vi "setpoint(SubVI).vi"(0 "Filed 2":dbl=300.0, 1 "Field":dbl=300.0, 2 "类型":enum16{"temp", "field", "position"}(ring), 3 "Rate/speed":dbl=10.0, 4 "Mode":i32(ring) items=["Persistent", "Driven"], 5 "输出簇 2":T1={"initialize"="", "6221"={"6221 Resource"="GPIB0::24::INSTR", "Delta status"=FALSE}, "7001"={"Ch"=FALSE}, "SR830+6221"={"source"=0, "阻抗"=0.0, "量程入 4"=0, "量程入 3"=0, "量程入 2"=0, "量程入 1"=0, "电流"=0.0, "SR830 2"=FALSE, "SR830 3"=FALSE, "SR830 4"=FALSE, "SR830 1"=FALSE, "VISA 1"="", "VISA 2"="", "VISA 3"="", "VISA 4"="", "量程"=enum."量程每次测量会判定"}, "2400"={"2400"=FALSE, "VISA"=""}, "ch"={"ch"=[], "current"=[], "change?"=[]}, "log"={"log路径"=path "", "log interval"=0.0}, "Instrument"={"335 Resource"="GPIB0::24::INSTR", "Input (0:A)"=0, "Instrument Type"=3, "quantum design"=refnum, "Heater Output (1:1)"=1, "semaphore"=refnum, "TCP master instance"=refnum, "335 Status"=refnum, "M24C Resource"="GPIB0::24::INSTR", "4G supply"="GPIB0::24::INSTR", "Temp Status 24C"=refnum, "4g supply status"=refnum}, "Aborting"=refnum, "数据文件"=refnum} {"Instrument"."Input (0:A)" items=["A", "B"]; "Instrument"."Instrument Type" items=["PPMS", "VersaLab", "DynaCool", "SVSM", "Lakeshore335", "PPMS-Rotate"]; "Instrument"."Heater Output (1:1)" items=["1"=1, "2"=2]; "SR830+6221"."source" items=["SR830 1", "SR830 2", "SR830 3", "SR830 4"]}, 6 "data":refnum<queue>, 7 "Delay":dbl, 9 "steps number":i32, 11 "Approach":i32(ring) items=["FastSettle", "NoOvershoot"]) -> (8 "错误输出":errorcluster, 15 "输出簇":T1={"initialize"="", "6221"={"6221 Resource"="GPIB0::24::INSTR", "Delta status"=FALSE}, "7001"={"Ch"=FALSE}, "SR830+6221"={"source"=0, "阻抗"=0.0, "量程入 4"=0, "量程入 3"=0, "量程入 2"=0, "量程入 1"=0, "电流"=0.0, "SR830 2"=FALSE, "SR830 3"=FALSE, "SR830 4"=FALSE, "SR830 1"=FALSE, "VISA 1"="", "VISA 2"="", "VISA 3"="", "VISA 4"="", "量程"=enum."量程每次测量会判定"}, "2400"={"2400"=FALSE, "VISA"=""}, "ch"={"ch"=[], "current"=[], "change?"=[]}, "log"={"log路径"=path "", "log interval"=0.0}, "Instrument"={"335 Resource"="GPIB0::24::INSTR", "Input (0:A)"=0, "Instrument Type"=3, "quantum design"=refnum, "Heater Output (1:1)"=1, "semaphore"=refnum, "TCP master instance"=refnum, "335 Status"=refnum, "M24C Resource"="GPIB0::24::INSTR", "4G supply"="GPIB0::24::INSTR", "Temp Status 24C"=refnum, "4g supply status"=refnum}, "Aborting"=refnum, "数据文件"=refnum} {"Instrument"."Input (0:A)" items=["A", "B"]; "Instrument"."Instrument Type" items=["PPMS", "VersaLab", "DynaCool", "SVSM", "Lakeshore335", "PPMS-Rotate"]; "Instrument"."Heater Output (1:1)" items=["1"=1, "2"=2]; "SR830+6221"."source" items=["SR830 1", "SR830 2", "SR830 3", "SR830 4"]})   [LabVIEW 2019, in "SubVI.lvlib"]
uses:
  SubVI.lvlib
  config.ctl
  <vilib>/NI/Modbus Library/API/Master/Modbus Master.lvclass
  Instrument.ctl
  lib/QDInstrument.dll
  335 state.ctl
  9T cmag.lvlib
panel:
  # "(真是通道1，假是通道2)"
  # "(真是通道1，假是通道2)"
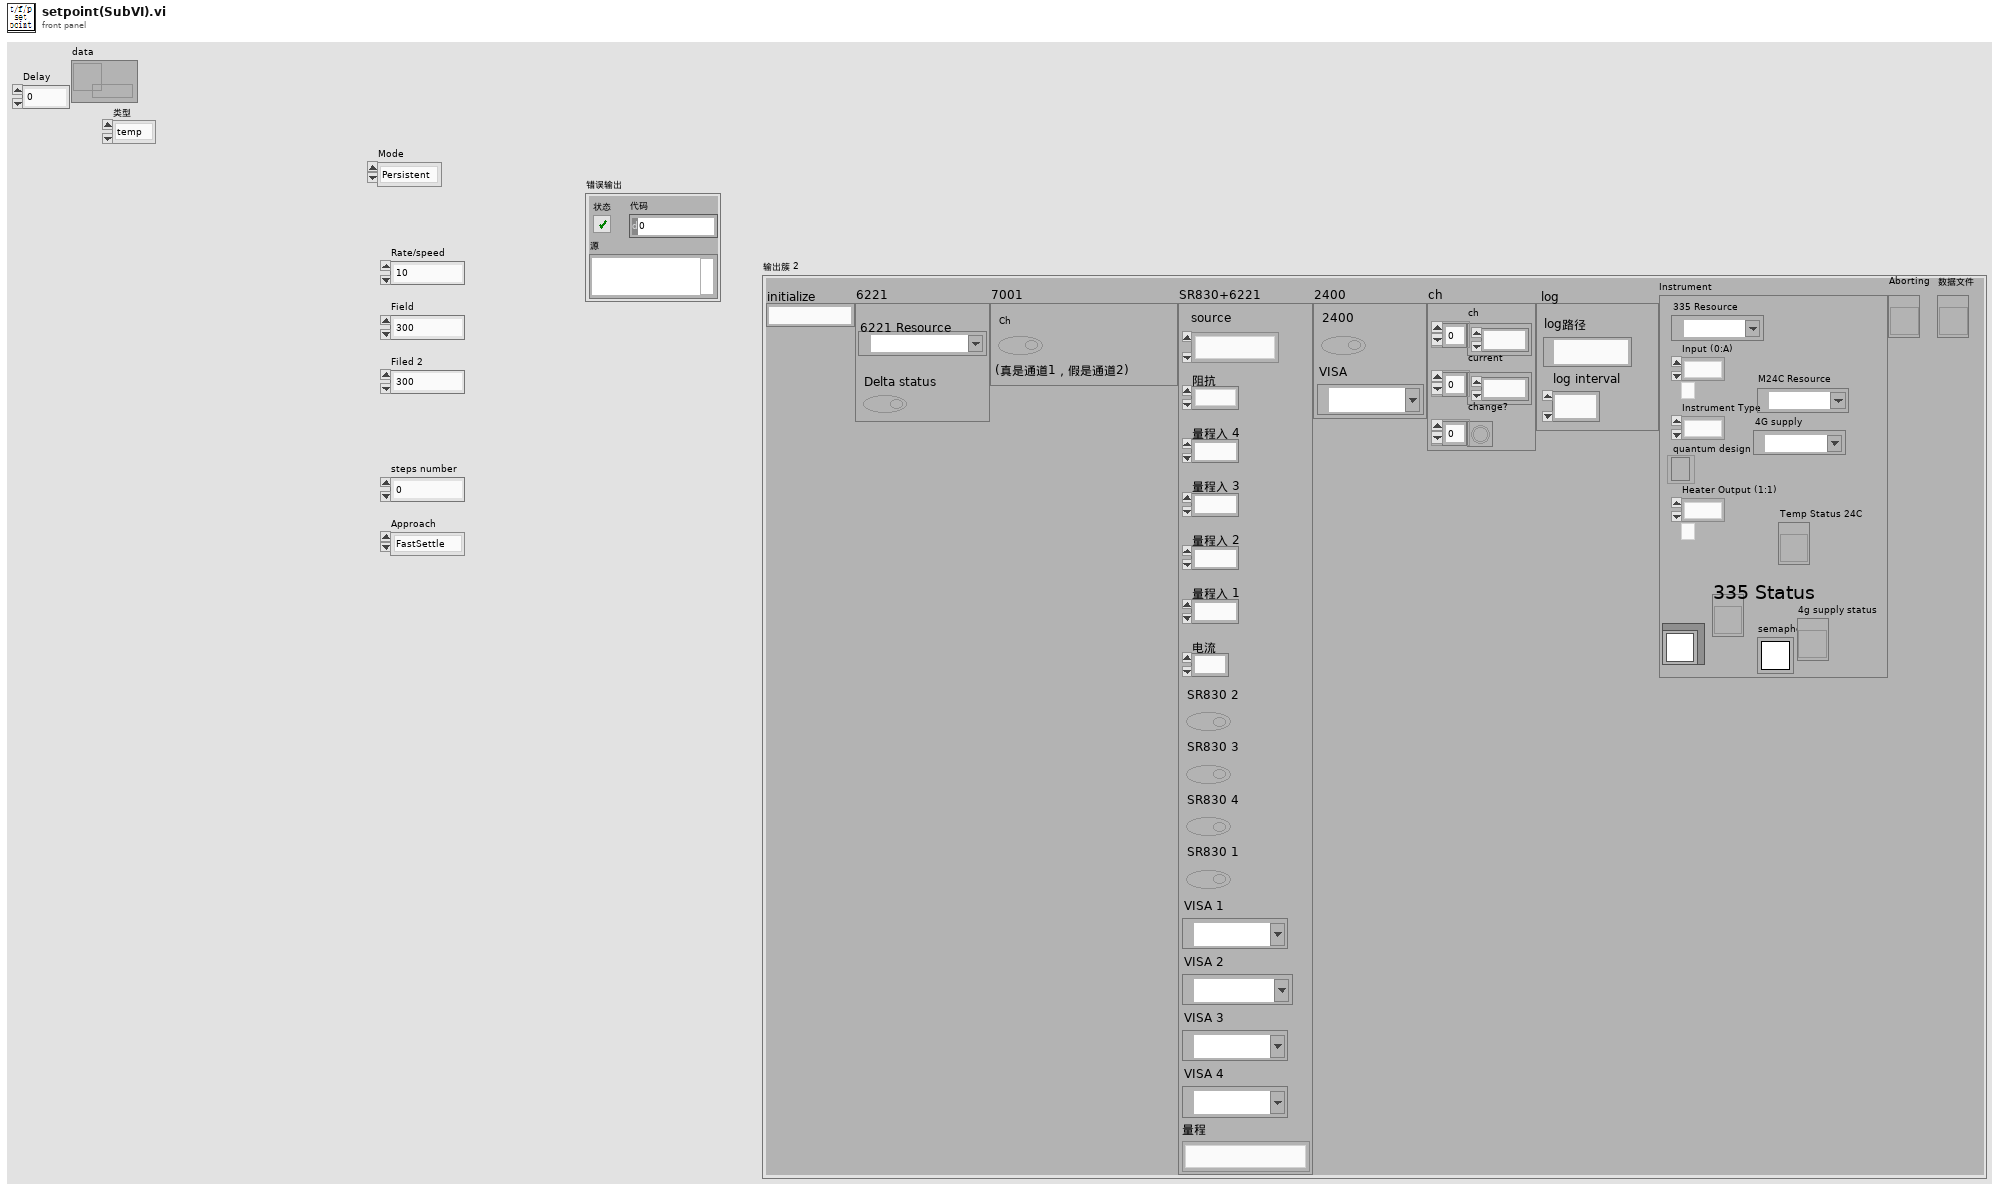
[diagram p1: front panel]
types:
  T1 = typedef "config.ctl" = cluster{"initialize":string, "6221":cluster{"6221 Resource":refnum<visa-resource-name>, "Delta status":bool}, "7001":cluster{"Ch":bool}, "SR830+6221":cluster{"source":u16, "阻抗":dbl, "量程入 4":i32, "量程入 3":i32, "量程入 2":i32, "量程入 1":i32, "电流":dbl, "SR830 2":bool, "SR830 3":bool, "SR830 4":bool, "SR830 1":bool, "VISA 1":refnum<visa-resource-name>, "VISA 2":refnum<visa-resource-name>, "VISA 3":refnum<visa-resource-name>, "VISA 4":refnum<visa-resource-name>, "量程":enum16{"量程每次测量会判定", "量程不变为设定值"}}, "2400":cluster{"2400":bool, "VISA":refnum<visa-resource-name>}, "ch":cluster{"ch":i32[], "current":dbl[], "change?":bool[]}, "log":cluster{"log路径":path, "log interval":dbl}, "Instrument":T2, "Aborting":refnum<vi>, "数据文件":refnum<vi>}
  T2 = typedef "Instrument.ctl" = cluster{"335 Resource":refnum<visa-resource-name>, "Input (0:A)":u16, "Instrument Type":i32, "quantum design":refnum<k24>, "Heater Output (1:1)":u16, "semaphore":T3, "TCP master instance":refnum<class "Modbus Master.lvclass">, "335 Status":refnum<vi>, "M24C Resource":refnum<visa-resource-name>, "4G supply":refnum<visa-resource-name>, "Temp Status 24C":refnum<vi>, "4g supply status":refnum<vi>}
  T3 = typedef "Semaphore RefNum" = refnum<k1>
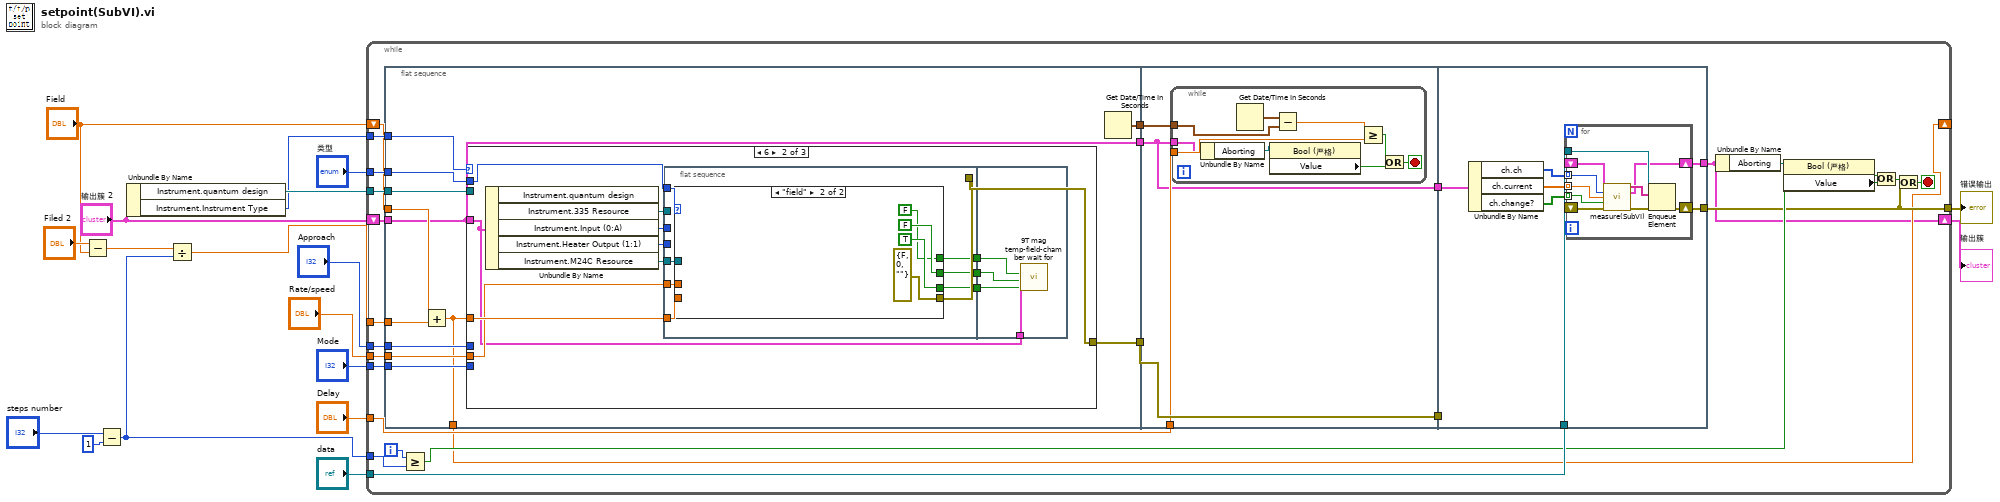
[diagram p0: block diagram]
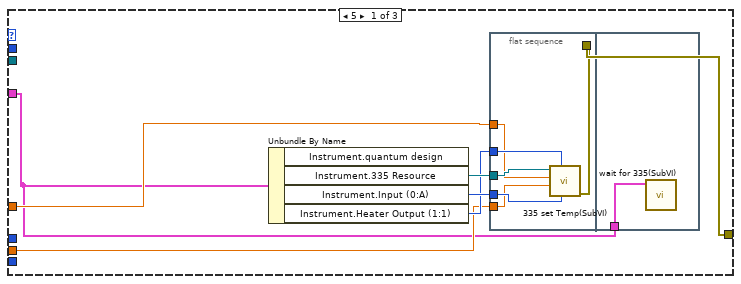
[diagram p2: hidden frame]
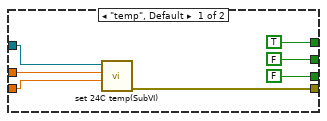
[diagram p3: hidden frame]
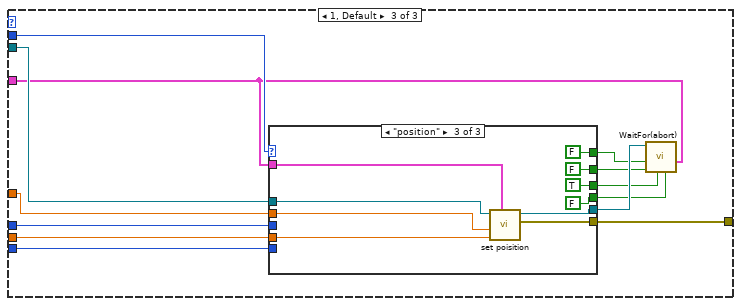
[diagram p4: hidden frame]
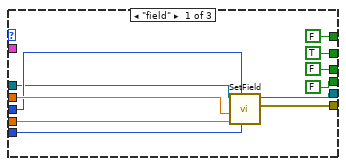
[diagram p5: hidden frame]
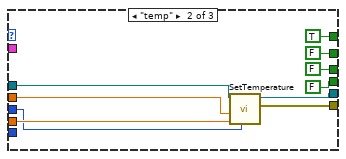
[diagram p6: hidden frame]
diagram:
  n1 = Subtract(x="Filed 2", y="Field") -> (x-y=w18:dbl)
  n2 = Subtract(x="steps number", y=1) -> (x-y=w10:i32)
  n3 = Unbundle By Name("输出簇 2") -> ("Instrument.quantum design"=w6:refnum<k24>, "Instrument.Instrument Type"=w5:i32)
  n4 = Divide(x=w18, y=w10) -> (x/y=w3:dbl)
  n5 = while {
    tunnel: w10 -> [w42]
    tunnel: "data" -> [w44]
    tunnel: "Mode" -> [w40]
    tunnel: "Approach" -> [w39]
    tunnel: "Rate/speed" -> [w38]
    tunnel: w6 -> [w37]
    tunnel: [w30] -> w13
    tunnel: "Delay" -> [w31]
    tunnel: "类型" -> [w29]
    tunnel: w5 -> [w28]
    shift-right: [w25] -> _
    shift-left: "Field" -> [w27]
    tunnel: w3 -> [w26]
    shift-right: [w21] -> w2
    shift-left: "输出簇 2" -> [w19]
    i -> [w41]
    stop <- w35 stop-if-true
    n6 = flat-sequence {
      tunnel: w40 -> [w56]
      tunnel: w39 -> [w55]
      tunnel: w38 -> [w54]
      tunnel: w37 -> [w53]
      tunnel: [w52] -> w34
      tunnel: [w51] -> w32
      tunnel: w29 -> [w50]
      tunnel: w28 -> [w49]
      tunnel: w27 -> [w48]
      tunnel: w26 -> [w47]
      tunnel: [w46] -> w25
      tunnel: w19 -> [w45]
      tunnel: [w45] -> w20
      tunnel: w34 -> [w153]
      tunnel: [w153] -> w33
      tunnel: w32 -> [w152]
      tunnel: w31 -> [w151]
      tunnel: [w150] -> w24
      tunnel: w20 -> [w150]
      tunnel: [w164] -> w30
      tunnel: w33 -> [_]
      tunnel: w44 -> [w165]
      tunnel: w24 -> [w169]
      tunnel: [w163] -> w21
      frame #0 {
        n7 = Add(x=w48, y=w47) -> (x+y=w46:dbl)
        n8 = case shown="6" w49 {
          tunnel: w46 -> [w60 w79 w118]
          tunnel: w56 -> [_ _ w117]
          tunnel: w55 -> [_ _ w116]
          tunnel: w54 -> [w59 w78 w115]
          tunnel: w53 -> [_ _ w114]
          tunnel: [w58 w77 w108] -> w52
          tunnel: w50 -> [_ w75 w107]
          tunnel: w45 -> [w57 w74 w106]
          frame 5 {
            n9 = Unbundle By Name(w57) -> ("Instrument.335 Resource"=w63:refnum<visa-resource-name>, "Instrument.Input (0:A)"=w62:u16, "Instrument.Heater Output (1:1)"=w61:u16)  [unwired: 1 out]
            n10 = flat-sequence {
              tunnel: w63 -> [w69]
              tunnel: w62 -> [w68]
              tunnel: w61 -> [w67]
              tunnel: w60 -> [w66]
              tunnel: w59 -> [w65]
              tunnel: [w64] -> w58
              tunnel: w57 -> [w70]
              frame #0 {
                n11 = call "335 set Temp(SubVI).vi"("Input (0:A)"=w68, "Output (1:1)"=w67, "Rate"=w65, "Temperature"=w66, "VISA Refnum in"=w69) -> ("error out"=w64:errorcluster)  [unwired: 5 in, 1 out]
              }
              frame #1 {
                n12 = call "wait for 335(SubVI).vi"("簇"=w70) -> ()  [unwired: 10 in]
              }
            }
          }
          frame 6 {
            n13 = Unbundle By Name(w74) -> ("Instrument.335 Resource"=w82:refnum<visa-resource-name>, "Instrument.Input (0:A)"=w81:u16, "Instrument.Heater Output (1:1)"=w80:u16, "Instrument.M24C Resource"=w76:refnum<visa-resource-name>)  [unwired: 1 out]
            n14 = flat-sequence {
              tunnel: w82 -> [_]
              tunnel: w81 -> [_]
              tunnel: w80 -> [_]
              tunnel: w79 -> [w88]
              tunnel: w78 -> [w89]
              tunnel: [w87] -> w77
              tunnel: w76 -> [w90]
              tunnel: w75 -> [w86]
              tunnel: [w85] -> w73
              tunnel: [w84] -> w72
              tunnel: [w83] -> w71
              tunnel: w74 -> [w105]
              tunnel: w73 -> [w104]
              tunnel: w72 -> [w103]
              tunnel: w71 -> [w102]
              frame #0 {
                n15 = case shown="\"field\"" w86 {
                  tunnel: w90 -> [w97 _]
                  tunnel: w89 -> [w96 _]
                  tunnel: w88 -> [w95 _]
                  tunnel: [w94 errorcluster {"status"=FALSE, "code"=0, "source"=""} ("ErrorOut")] -> w87
                  tunnel: [FALSE ("Field") TRUE ("Field")] -> w85
                  tunnel: [FALSE ("Chamber") FALSE ("Chamber")] -> w84
                  tunnel: [TRUE ("temp") FALSE ("temp")] -> w83
                  frame "temp", Default {
                    n16 = call "set 24C temp(SubVI).vi"("Temperature"=w95, "Rate"=w96, "VISA引用句柄输入"=w97) -> ("ErrorOut"=w94:errorcluster)  [unwired: 8 in]
                  }
                  frame "field" {
                  }
                }
              }
              frame #1 {
                n17 = call "9T mag temp-field-chamber wait for.vi"("Field"=w104, "Chamber"=w103, "temp"=w102, "输出簇"=w105) -> ()  [unwired: 8 in]
              }
            }
          }
          frame 1, Default {
            n18 = case shown="\"position\"" w107 {
              tunnel: w118 -> [w129 w134 w142]
              tunnel: w117 -> [w128 _ _]
              tunnel: w116 -> [w127 w132 _]
              tunnel: w115 -> [w126 w133 w141]
              tunnel: w114 -> [w125 w135 w145]
              tunnel: [w124 w131 w144] -> w113
              tunnel: [FALSE ("Wait For Temperature") TRUE ("Wait For Temperature") FALSE ("Wait For Temperature")] -> w112
              tunnel: [TRUE ("Wait For Field") FALSE ("Wait For Field") FALSE ("Wait For Field")] -> w111
              tunnel: [FALSE ("Wait For Position") FALSE ("Wait For Position") TRUE ("Wait For Position")] -> w110
              tunnel: [FALSE ("Wait For Chamber") FALSE ("Wait For Chamber") FALSE ("Wait For Chamber")] -> w109
              tunnel: [w119 w130 w143] -> w108
              tunnel: w106 -> [_ _ w140]
              frame "field" {
                n19 = call "SetField.vi"("Mode"=w128, "Approach"=w127, "Rate"=w126, "Field"=w129, "Instrument Ref In"=w125) -> ("error out"=w119:errorcluster, "Instrument Ref Out"=w124:refnum<k24>)  [unwired: 2 in, 1 out]
              }
              frame "temp" {
                n20 = call "SetTemperature.vi"("Approach"=w132, "Rate"=w133, "Temperature"=w134, "Instrument Ref In"=w135) -> ("error out"=w130:errorcluster, "Instrument Ref Out"=w131:refnum<k24>)  [unwired: 3 in, 1 out]
              }
              frame "position" {
                n21 = call "set poisition.vi"("簇"=w140, "Slow down code\ndefault = 0"=w141, "Position (deg)"=w142, "Instrument Ref In"=w145) -> ("error out"=w143:errorcluster, "Instrument Ref Out"=w144:refnum<k24>)  [unwired: 4 in]
              }
            }
            n22 = call "WaitFor(abort).vi"("簇"=w106, "Wait For Chamber"=w109, "Wait For Position"=w110, "Wait For Field"=w111, "Wait For Temperature"=w112, "Instrument Ref In"=w113) -> ()  [unwired: 4 in, 2 out]
          }
        }
        n23 = Get Date/Time In Seconds() -> (seconds since 1Jan1904=w51:timestamp)
      }
      frame #1 {
        n24 = while {
          tunnel: w152 -> [w161]
          tunnel: w151 -> [w159]
          tunnel: w150 -> [w156]
          stop <- w157 stop-if-true
          n25 = Unbundle By Name(w156) -> ("Aborting"=w155:refnum<vi>)
          n26 = Get Date/Time In Seconds() -> (seconds since 1Jan1904=w162:timestamp)
          n27 = property class="Bool (严格)"(reference=w155) -> ("Value"=w154:bool)  [unwired: 1 in, 2 out]
          n28 = Subtract(x=w162, y=w161) -> (x-y=w160:dbl)
          n29 = Greater Or Equal?(x=w160, y=w159) -> (x >= y?=w158:bool)
          n30 = Or(x=w158, y=w154) -> (x .or. y?=w157:bool)
        }
      }
      frame #2 {
        n31 = Unbundle By Name(w169) -> ("ch.ch"=w168:i32[], "ch.current"=w167:dbl[], "ch.change?"=w166:bool[])
        n32 = for {
          tunnel: w168 -> [w177] mode=indexing
          tunnel: w166 -> [w175] mode=indexing
          tunnel: w167 -> [w176] mode=indexing
          tunnel: w165 -> [w179]
          shift-right: [w173] -> w163
          shift-left: _ -> [w178]
          shift-right: [w170] -> w164
          shift-left: _ -> [w172]
          n33 = call "measure(SubVI).vi"("config in"=w178, "ch"=w177, "current"=w176, "change?"=w175, "error in (no error)"=w172) -> ("data"=w174:string[], "config out"=w173:T1, "error out"=w171:errorcluster)  [unwired: 8 in]
          n34 = Enqueue Element(queue=w179, element=w174, error in (no error)=w171) -> (error out=w170:errorcluster)  [unwired: 1 in, 2 out]
        }
      }
    }
    n35 = Greater Or Equal?(x=w41, y=w42) -> (x >= y?=w43:bool)
    n36 = Unbundle By Name(w21) -> ("Aborting"=w23:refnum<vi>)
    n37 = property class="Bool (严格)"(reference=w23) -> ("Value"=w22:bool)  [unwired: 1 in, 2 out]
    n38 = Or(x=w43, y=w22) -> (x .or. y?=w36:bool)
    n39 = Or(x=w36, y=w30) -> (x .or. y?=w35:bool)
  }
  "错误输出" <- w13
  "输出簇" <- w2
